vi "LoadPiezoTrajactory.vi"(1 "Z backforth 采样信息":cluster{"采样率":dbl, "采样数":dbl}={"采样率"=500000.0, "采样数"=400000.0}, 2 "File Sampling Rate":dbl=1000.0, 3 "Path":path=path "D:/APP/LightSheetController_Ver8 obl/VISource/Waveform/Piezo_feedback_20201106.txt") -> (0 "output waveform":waveform(dbl)(graph))   [LabVIEW 2018]
uses:
  <vilib>/measure/maresamp.llb/Resample Waveform (single shot).vi
  <vilib>/measure/NI_MAPro.lvlib
panel:
  out "size(s)":i32
  out "element":dbl
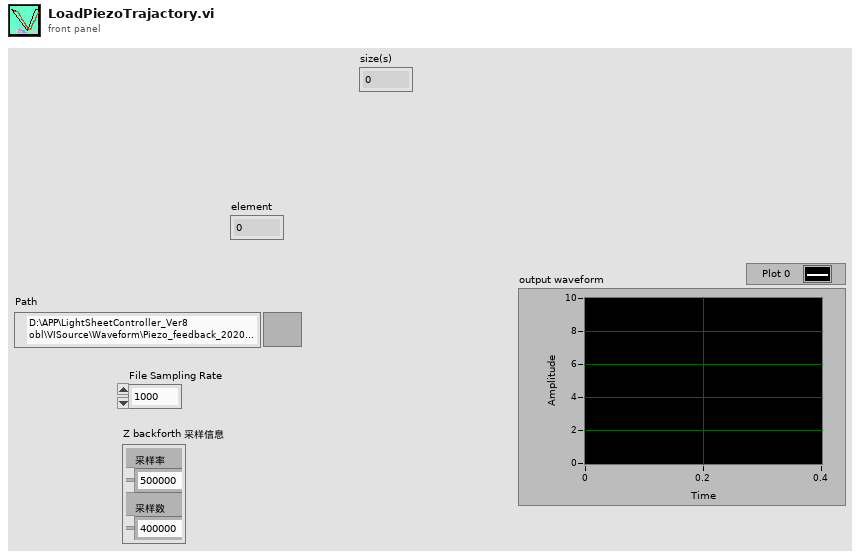
[diagram p1: front panel]
types:
  T1 = cluster{"alias rejection (dB)":dbl, "normalized bandwidth":dbl}
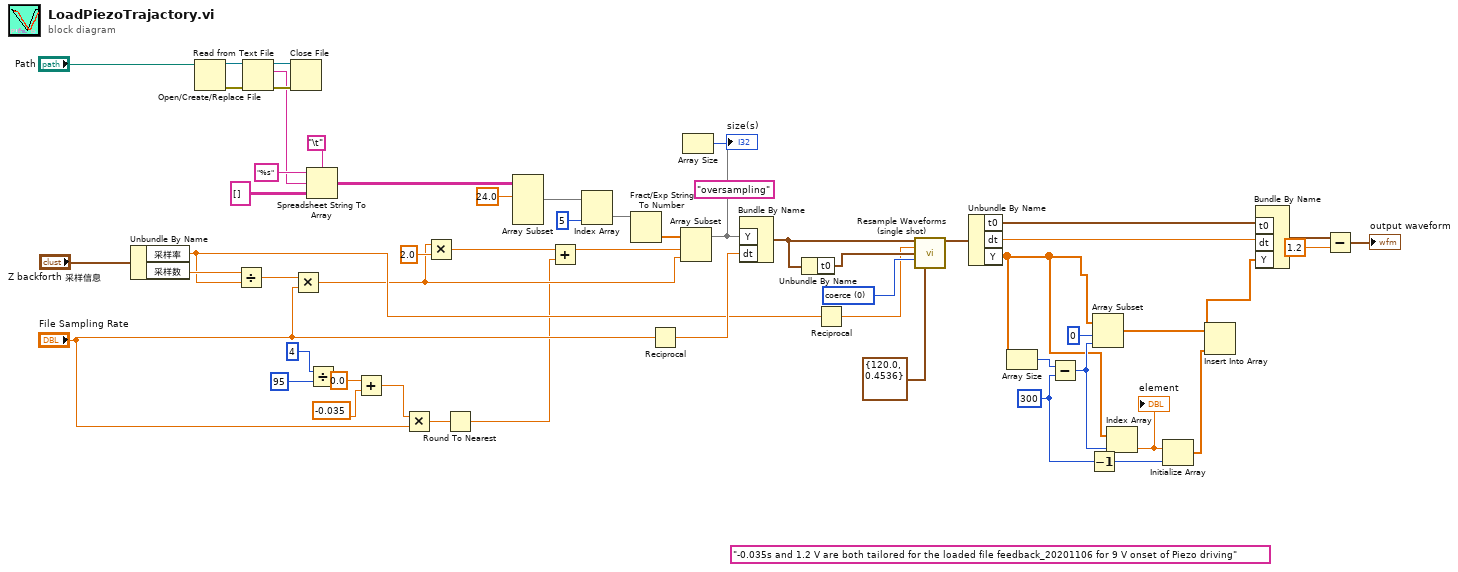
[diagram p0: block diagram]
diagram:
  (unwired) "-0.035s and 1.2 V are both tailored for the loaded file feedback_20201106 for 9 V onset of Piezo driving"
  w28 = 300 ("y")
  w34 = u16 0 items=["coerce", "linear", "spline", "FIR filter"] ("interpolation mode")
  (unwired) "oversampling"
  n1 = Unbundle By Name("Z backforth 采样信息") -> ("采样率"=w21:dbl, "采样数"=w38:dbl)
  n2 = Open/Create/Replace File(file path (use dialog)="Path") -> (refnum out=w47:refnum<file>, error out=w50:errorcluster)  [unwired: 5 in, 1 out]
  n3 = Divide(x=w38, y=w21) -> (x/y=w37:dbl)
  n4 = Read from Text File(file (use dialog)=w47, error in=w50) -> (refnum out=w48:refnum<file>, text=w42:string, error out=w49:errorcluster)  [unwired: 2 in, 1 out]
  n5 = Close File(refnum=w48, error in=w49) -> ()  [unwired: 2 out]
  n6 = Multiply(x=w37, y="File Sampling Rate") -> (x*y=w9:dbl)
  n7 = Spreadsheet String To Array(delimiter (Tab)="\t", format string="%s" ("spreadsheet string"), spreadsheet string=w42, array type (2D Dbl)=string[][] []) -> (array=w44:string[][])
  n8 = Divide(x=4 ("index"), y=95) -> ()  [unwired: 1 out]
  n9 = Add(x=0.0, y=-0.035) -> (x+y=w5:dbl)
  n10 = Multiply(x=w5, y="File Sampling Rate") -> (x*y=w13:dbl)
  n11 = Multiply(x=w9, y=2.0) -> (x*y=w10:dbl)
  n12 = Round To Nearest(number=w13) -> (nearest integer value=w7:dbl)
  n13 = Array Subset(array=w44, index (row)=24.0 ("y")) -> (w53:string[][])  [unwired: 3 in]
  n14 = Add(x=w10, y=w7) -> (x+y=w8:dbl)
  n15 = Index Array(array=w53, index (col)=5 ("disabled index (col)")) -> (element=w54:string[])  [unwired: 1 in]
  n16 = Fract/Exp String To Number(string=w54) -> (number=w15:dbl[])  [unwired: 3 in, 1 out]
  n17 = Reciprocal(x="File Sampling Rate") -> (1/x=w41:dbl)
  n18 = Array Subset(array=w15, index=w8, length=w9) -> (w11:dbl[])
  n19 = Array Size(array=w11) -> (size(s)=→"size(s)":i32)
  n20 = Bundle By Name("Y"=w11, "dt"=w41) -> (w36:waveform(dbl))  [unwired: 1 in]
  n21 = Unbundle By Name(w36) -> ("t0"=w35:timestamp)
  n22 = Reciprocal(x=w21) -> (1/x=w32:dbl)
  n23 = call-poly <vilib>:"Resample Waveforms (single shot).vi"("waveform in"=w36, "dt"=w32, "t0"=w35, "interpolation mode"=w34, "FIR filter specifications"=T1 {"alias rejection (dB)"=120.0, "normalized bandwidth"=0.4536}) -> ("resampled waveform out"=w16:waveform(dbl))  [unwired: 7 in, 3 out]
  n24 = Unbundle By Name(w16) -> ("t0"=w31:timestamp, "dt"=w30:dbl, "Y"=w18:dbl[])
  n25 = Array Size(array=w18) -> (size(s)=w22:i32)
  n26 = Subtract(x=w22, y=w28) -> (x-y=w27:i32)
  n27 = Decrement(x=w28) -> (x-1=w23:i32)
  n28 = Array Subset(array=w18, index=0, length=w27) -> (w25:dbl[])
  n29 = Index Array(array=w18, index=w27) -> (element=w26:dbl)
  "element" <- w26
  n30 = Initialize Array(w26, w23) -> (w24:dbl[])
  n31 = Insert Into Array(array=w25, new element=w24) -> (w19:dbl[])  [unwired: 1 in]
  n32 = Bundle By Name("t0"=w31, "dt"=w30, "Y"=w19) -> (w3:waveform(dbl))  [unwired: 1 in]
  n33 = Subtract(x=w3, y=1.2) -> (x-y=→"output waveform":waveform(dbl))
